vi "Requests.vi"(8 "error in (no error)":errorcluster, 9 "write enable":bool=TRUE, 11 "ICPCON ET in":refnum<class "NS300.lvclass">) -> (0 "error out":errorcluster, 3 "ICPCON ET out":refnum<class "NS300.lvclass">)   [LabVIEW 2019, in "NS300.lvclass"]
uses:
  NS300.lvclass
  C:/my_projects/projects/Algorithms/Labview/19/Modbus/MB_TCP2/MB_TCP.lvclass
  MB_TCP.lvclass/MB_TCP.ctl
  NI_modbus_upd/Ctl/Unit_ID.ctl
  NI_modbus_upd/TCP/TCP.lvclass/TCP.ctl
  NI_modbus_upd/Function data mismatch error1.vi
  NI_modbus_upd/Master Function Definition/Responses/Write Multiple Registers Response.vi
  NI_modbus_upd/Master Function Definition/Requests/Write Multiple Registers Request.vi
  NI_modbus_upd/Master network read write.vi
  NI_modbus_upd/Master Function Definition/Responses/Read Input Registers Response.vi
  NI_modbus_upd/Master Function Definition/Requests/Read Input Registers Request.vi
  NI_modbus_upd/Master Function Definition/Responses/Read Holding Registers Response.vi
  NI_modbus_upd/Master Function Definition/Requests/Read Holding Registers Request.vi
  NI_modbus_upd/Function code mismatch error1.vi
  NI_modbus_upd/Error Generator1.vi
  NI_modbus_upd/Modbus Data Unit (PDU)/Construct PDU1.vi
  NI_modbus_upd/Utility/U16s to Bytes1.vi
  NI_modbus_upd/Read ADU Packet Master.vi
  NI_modbus_upd/Write ADU Packet Master.vi
  NI_modbus_upd/Utility/Bytes to U16s1.vi
  NI_modbus_upd/Modbus Data Unit (PDU)/Unflatten to PDU1.vi
  NI_modbus_upd/TCP/Protocol Read.vi
  NI_modbus_upd/TCP/Protocol Write.vi
  <vilib>/Utility/error.llb/Clear Errors.vi
  NI_modbus_upd/Modbus Data Unit (PDU)/Deconstruct PDU1.vi
  NI_modbus_upd/TCP/TCP.lvclass
  ICPCON Registers/ICPCON Registers.lvlib
  MB_TCP.lvclass
  NI_modbus_upd/NI_modbus_upd.lvlib
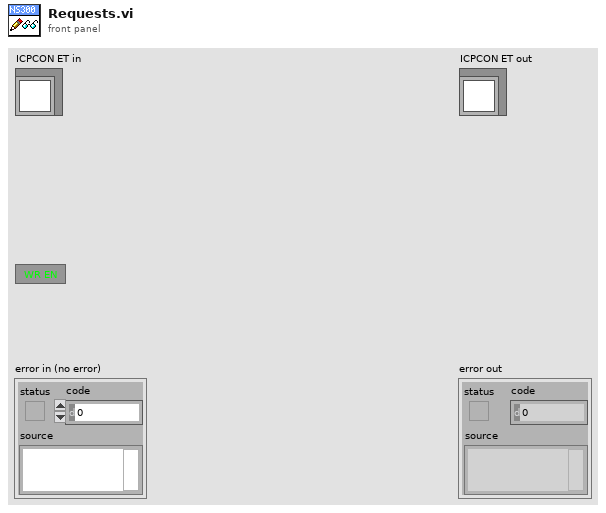
[diagram p1: front panel]
types:
  T1 = typedef "NI_modbus_upd.lvlib/Unit_ID.ctl" = cluster{"Protocol ID":u16, "Unit ID":u8}
  T2 = typedef "ICPCON Registers.lvlib/ICPCON Data.ctl" = cluster{"UTF":refnum<data-value>, "DI":refnum<data-value>, "DW":refnum<data-value>, "DO":refnum<data-value>, "IR":refnum<data-value>, "WR":refnum<data-value>, "OR":refnum<data-value>, "modified":refnum<data-value>}
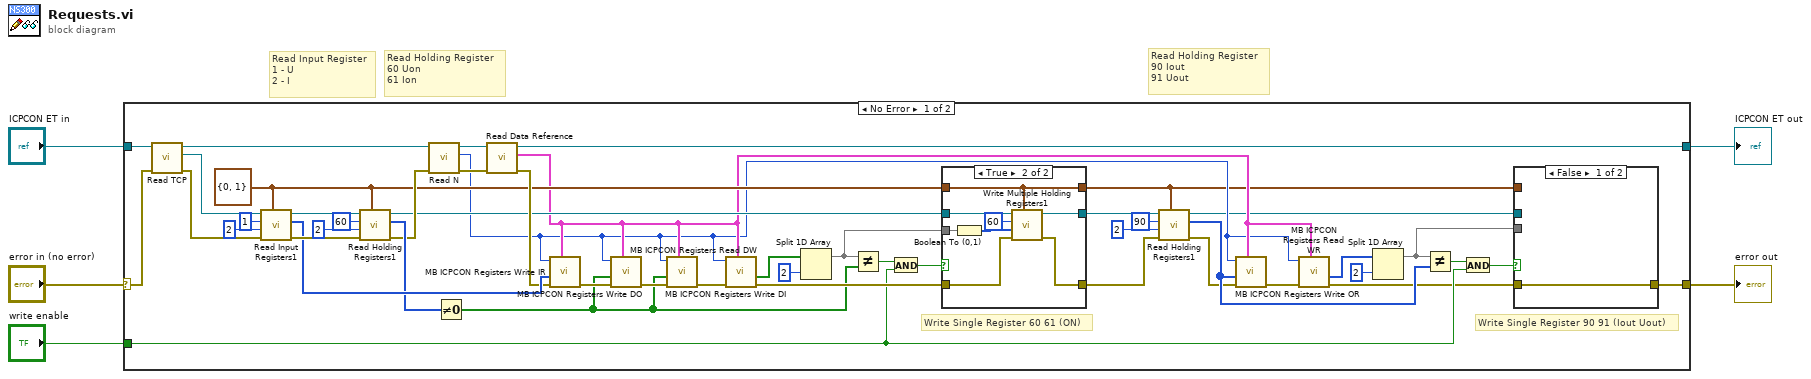
[diagram p0: block diagram]
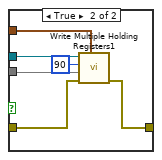
[diagram p2: hidden frame]
diagram:
  # "Read Holding Register\n90 Iout\n91 Uout"
  # "Read Holding Register\n60 Uon\n61 Ion"
  # "Read Input Register\n1 - U\n2 - I"
  n1 = case shown="No Error" "error in (no error)" {
    selector: "error in (no error)" -> [w36 w74]
    tunnel: [w6 w74] -> w3
    tunnel: [w7 w73] -> w4
    tunnel: "ICPCON ET in" -> [w37 w73]
    tunnel: "write enable" -> [w38 _]
    frame No Error {
      w21 = T1 {"Protocol ID"=0, "Unit ID"=1} ("Unit_ID")
      # "Write Single Register 90 91 (Iout Uout)"
      # "Write Single Register 60 61 (ON)"
      n2 = call "Read TCP.vi"("error in (no error)"=w36, "MB_TCP in"=w37) -> ("error out"=w33:errorcluster, "TCP"=w34:refnum<class "TCP.lvclass">, "MB_TCP out"=w26:refnum<class "NS300.lvclass">)  [unwired: 7 in]
      n3 = call "Read Input Registers1.vi"("Unit_ID"=w21, "error in (no error)"=w33, "number of input registers"=u16 2, "starting address"=u16 1, "Modbus master in"=w34) -> ("error out"=w30:errorcluster, "register values"=w27:u16[], "Modbus master out"=w35:refnum<class "TCP.lvclass">)  [unwired: 4 in]
      n4 = call "Read Holding Registers1.vi"("Unit_ID"=w21, "error in (no error)"=w30, "number of holding registers"=u16 2, "starting address"=u16 60, "Modbus master in"=w35) -> ("error out"=w24:errorcluster, "register values"=w25:u16[], "Modbus master out"=w22:refnum<class "TCP.lvclass">)  [unwired: 4 in]
      n5 = call "Read N.vi"("error in (no error)"=w24, "MB_TCP in"=w26) -> ("error out"=w54:errorcluster, "N"=w13:i32, "MB_TCP out"=w53:refnum<class "NS300.lvclass">)  [unwired: 7 in]
      n6 = Not Equal To 0?(x=w25) -> (x != 0?=w39:bool[])
      n7 = call "Read Data Reference.vi"("error in (no error)"=w54, "MB_TCP in"=w53) -> ("error out"=w23:errorcluster, "Data"=w14:T2, "MB_TCP out"=w7:refnum<class "NS300.lvclass">)  [unwired: 7 in]
      n8 = call "MB ICPCON Registers Write IR.vi"("Data Reference"=w14, "error in (no error)"=w23, "Words In"=w27, "N"=w13) -> ("error out"=w52:errorcluster)  [unwired: 7 in]
      n9 = call "MB ICPCON Registers Write DO.vi"("Data Reference"=w14, "error in (no error)"=w52, "Bits In"=w39, "N"=w13) -> ("error out"=w41:errorcluster)  [unwired: 7 in]
      n10 = call "MB ICPCON Registers Write DI.vi"("Data Reference"=w14, "error in (no error)"=w41, "Bits In"=w39, "N"=w13) -> ("error out"=w40:errorcluster)  [unwired: 7 in]
      n11 = call "MB ICPCON Registers Read DW.vi"("Data Reference"=w14, "error in (no error)"=w40, "N"=w13) -> ("error out"=w46:errorcluster, "Bits out"=w49:bool[])  [unwired: 7 in]
      n12 = Split 1D Array(array=w49, index=2 ("length")) -> (first subarray=w47:bool[])  [unwired: 1 out]
      n13 = Not Equal?(x=w47, y=w39) -> (x != y?=w51:bool)
      n14 = And(x=w51, y=w38) -> (x .and. y?=w50:bool)
      n15 = case shown="True" w50 {
        tunnel: w46 -> [w64 w70]
        tunnel: [w64 w67] -> w16
        tunnel: w47 -> [_ w72]
        tunnel: w22 -> [w63 w71]
        tunnel: w21 -> [w62 w65]
        tunnel: [w63 w66] -> w18
        tunnel: [w62 w65] -> w10
        frame False {
        }
        frame True {
          n16 = Boolean To (0,1)(Boolean=w72) -> (0, 1=w69:i16[])
          n17 = call "Write Multiple Holding Registers1.vi"("Unit_ID"=w65, "error in (no error)"=w70, "holding register values"=w69, "starting address"=u16 60, "Modbus master in"=w71) -> ("error out"=w67:errorcluster, "Modbus master out"=w66:refnum<class "TCP.lvclass">)  [unwired: 5 in]
        }
      }
      n18 = call "Read Holding Registers1.vi"("Unit_ID"=w10, "error in (no error)"=w16, "number of holding registers"=u16 2, "starting address"=u16 90, "Modbus master in"=w18) -> ("error out"=w15:errorcluster, "register values"=w17:u16[], "Modbus master out"=w9:refnum<class "TCP.lvclass">)  [unwired: 4 in]
      n19 = call "MB ICPCON Registers Write OR.vi"("Data Reference"=w14, "error in (no error)"=w15, "Words In"=w17, "N"=w13) -> ("error out"=w43:errorcluster)  [unwired: 7 in]
      n20 = call "MB ICPCON Registers Read WR.vi"("Data Reference"=w14, "error in (no error)"=w43, "N"=w13) -> ("error out"=w8:errorcluster, "Words out"=w44:u16[])  [unwired: 7 in]
      n21 = Split 1D Array(array=w44, index=2 ("length")) -> (first subarray=w11:u16[])  [unwired: 1 out]
      n22 = Not Equal?(x=w11, y=w17) -> (x != y?=w42:bool)
      n23 = And(x=w42, y=w38) -> (x .and. y?=w12:bool)
      n24 = case shown="False" w12 {
        tunnel: w8 -> [w55 w60]
        tunnel: [w55 w58] -> w6
        tunnel: w9 -> [_ w61]
        tunnel: w10 -> [_ w57]
        tunnel: w11 -> [_ w56]
        frame False {
        }
        frame True {
          n25 = call "Write Multiple Holding Registers1.vi"("Unit_ID"=w57, "error in (no error)"=w60, "holding register values"=w56, "starting address"=u16 90, "Modbus master in"=w61) -> ("error out"=w58:errorcluster)  [unwired: 5 in, 1 out]
        }
      }
    }
    frame Error {
    }
  }
  "error out" <- w3
  "ICPCON ET out" <- w4
